vi "Bool Long Konvertierung.vi"(10 "Numerisch":i32, 11 "ES_BOOL":bool) -> (2 "ES_BOOL":bool, 3 "Numerisch":i32)   [LabVIEW 2017]
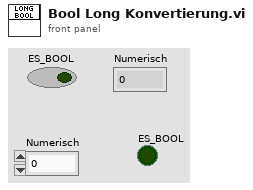
[diagram p1: front panel]
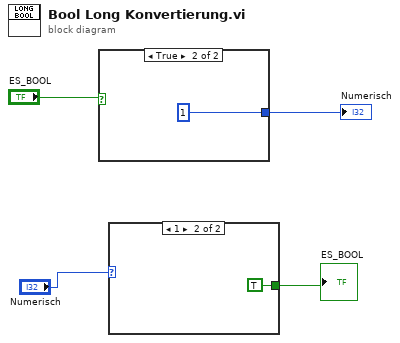
[diagram p0: block diagram]
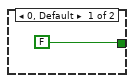
[diagram p2: hidden frame]
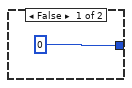
[diagram p3: hidden frame]
diagram:
  n1 = case shown="True" "ES_BOOL" {
    tunnel: [0 1] -> w4
    frame False {
    }
    frame True {
    }
  }
  "Numerisch" <- w4
  n2 = case shown="1" "Numerisch" {
    tunnel: [FALSE TRUE] -> w1
    frame 0, Default {
    }
    frame 1 {
    }
  }
  "ES_BOOL" <- w1
